vi "BindPropertyToRegister.vi"(9 "context":string, 10 "properties":T1[](array[typedef]), 11 "registers":T2[](array[typedef])) -> (3 "registers":T2[](array[typedef]))   [LabVIEW 2018, in "Paser.lvlib"]
uses:
  Paser.lvlib
  Ctrl/Register.ctl
  Ctrl/Bitfield.ctl
  Ctrl/Property.ctl
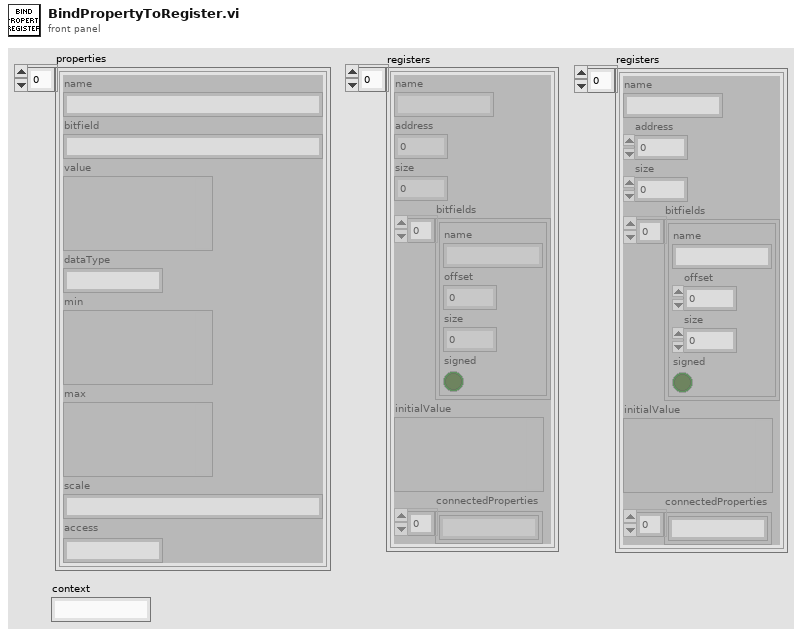
[diagram p1: front panel]
types:
  T1 = typedef "Property.ctl" = cluster{"name":string, "bitfield":string, "value":variant, "dataType":string, "min":variant, "max":variant, "scale":string, "access":string}
  T2 = typedef "Register.ctl" = cluster{"name":string, "address":i32, "size":i32, "bitfields":T3[], "initialValue":variant, "connectedProperties":string[]}
  T3 = typedef "Bitfield.ctl" = cluster{"name":string, "offset":i32, "size":i32, "signed":bool}
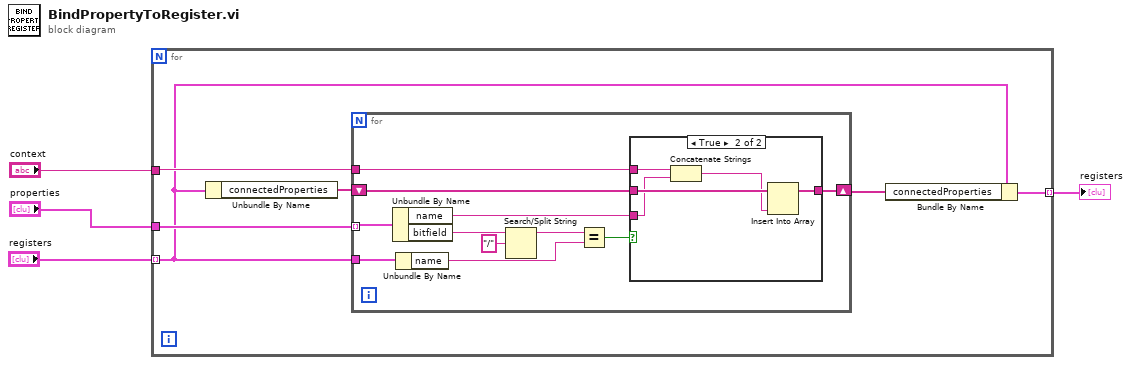
[diagram p0: block diagram]
diagram:
  n1 = for {
    tunnel: "properties" -> [w10]
    tunnel: "registers" -> [w6] mode=indexing
    tunnel: [w8] -> w3 mode=indexing
    tunnel: "context" -> [w7]
    n2 = Unbundle By Name(w6) -> ("connectedProperties"=w5:string[])
    n3 = for {
      tunnel: w6 -> [w18]
      tunnel: w10 -> [w21] mode=indexing
      shift-right: [w12] -> w9
      shift-left: w5 -> [w14]
      tunnel: w7 -> [w11]
      n4 = Unbundle By Name(w21) -> ("name"=w13:string, "bitfield"=w20:string)
      n5 = Unbundle By Name(w18) -> ("name"=w16:string)
      n6 = Search/Split String(string=w20, search string/char (-)="/") -> (substring before match=w17:string)  [unwired: 1 in, 2 out]
      n7 = Equal?(x=w17, y=w16) -> (x = y?=w15:bool)
      n8 = case shown="True" w15 {
        tunnel: w14 -> [w22 w27]
        tunnel: w13 -> [_ w24]
        tunnel: [w22 w26] -> w12
        tunnel: w11 -> [_ w25]
        frame False {
        }
        frame True {
          n9 = Concatenate Strings(w25, w24) -> (w23:string)
          n10 = Insert Into Array(array=w27, new element=w23) -> (w26:string[])  [unwired: 1 in]
        }
      }
    }
    n11 = Bundle By Name(cluster=w6, "connectedProperties"=w9) -> (w8:T2)
  }
  "registers" <- w3
